vi "Get_Day_File_Data.vi"(4 "Use Full Res Files":bool, 5 "Averaging Time (min)":dbl=5.0, 6 "End time":timestamp, 7 "Start time":timestamp, 8 "Channel Names":string[](array[string])=["EnFlo Tun:Usonic Fixed:Velocity"], 9 "Data folder location":path) -> (0 "Files with wrong times":path[](array[path]), 1 "All Channel Names":string[](array[string]), 2 "Data":dbl[][](array[numeric]), 3 "Times":dbl[](array[numeric]))   [LabVIEW 2020]
uses:
  Anemometry/Anemometry Sub Vis/Globals/Constants_global.vi
  Anemometry/Anemometry Sub Vis/Globals/Preference_global.vi
panel:
  out "Currenly reading":path
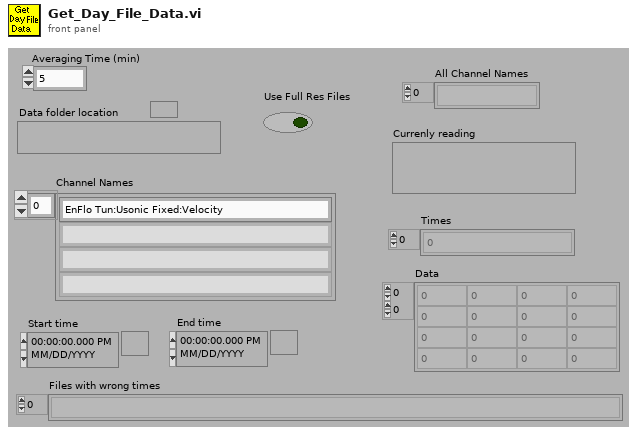
[diagram p1: front panel]
types:
  T1 = typedef "LVDateTimeRec.ctl" = cluster{"fractional second":dbl, "second":i32, "minute":i32, "hour":i32, "day of month":i32, "month":i32, "year":i32, "day of week":i32, "day of year":i32, "DST":i32}
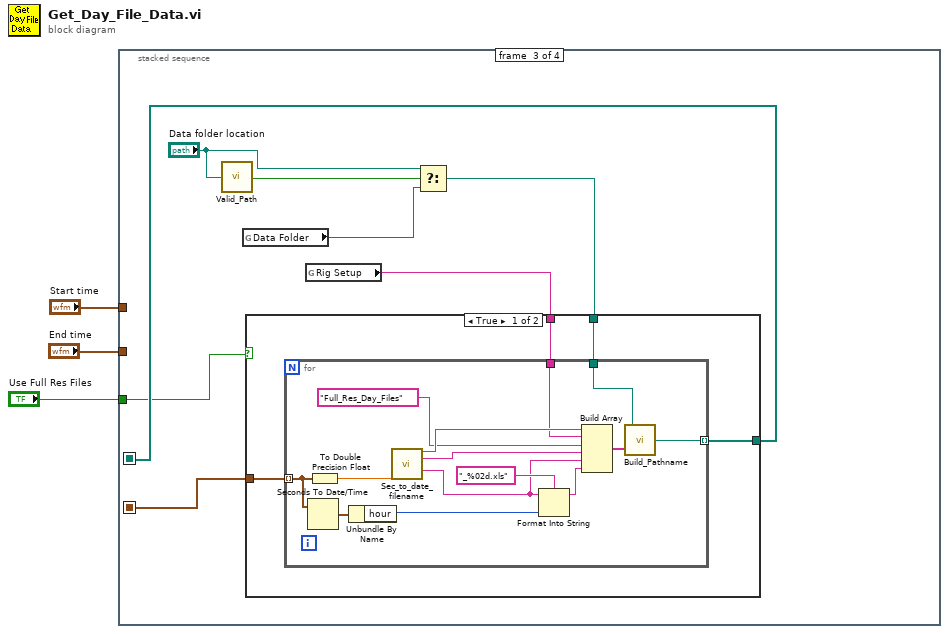
[diagram p0: block diagram]
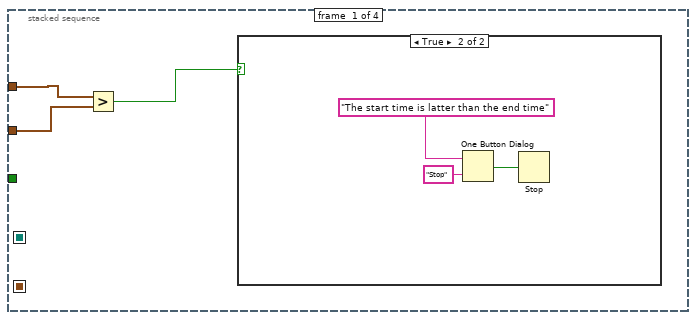
[diagram p2: hidden frame]
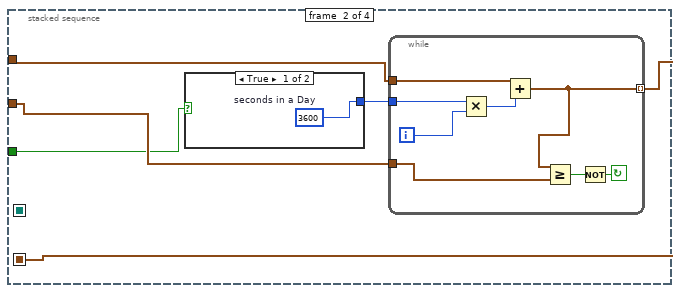
[diagram p4: hidden frame]
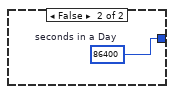
[diagram p5: hidden frame]
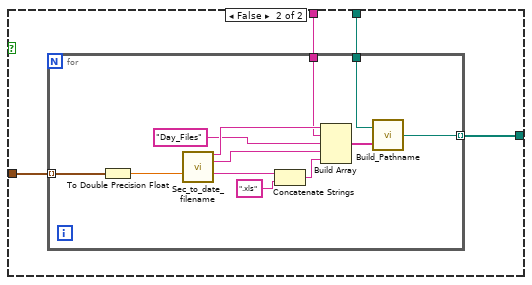
[diagram p6: hidden frame]
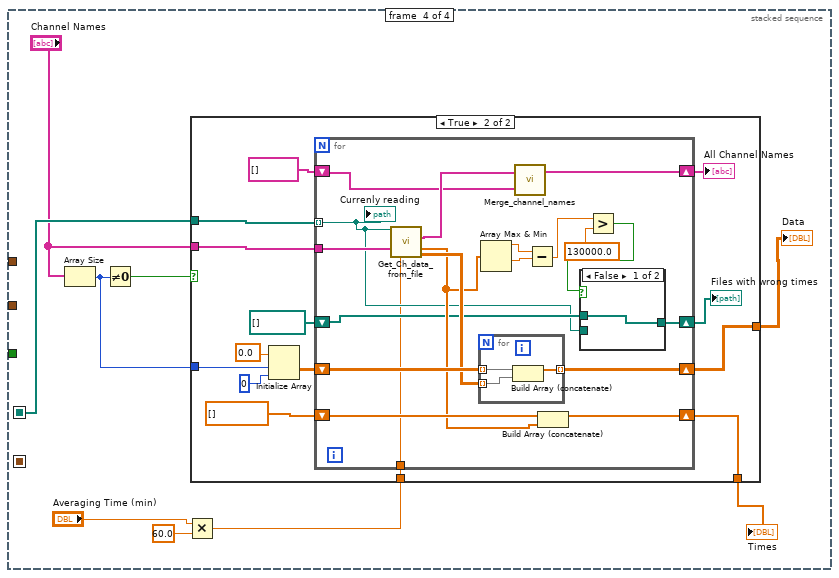
[diagram p7: hidden frame]
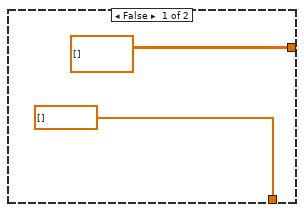
[diagram p8: hidden frame]
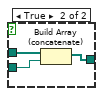
[diagram p9: hidden frame]
diagram:
  n1 = stacked-sequence {
    seq-local: [_ w14 _ _] -> [_ _ w32 _]
    seq-local: [_ _ w31 _] -> [_ _ _ w75]
    tunnel: "End time" -> [w5 w11 _ _]
    tunnel: "Start time" -> [w4 w12 _ _]
    tunnel: "Use Full Res Files" -> [_ w10 w25 _]
    frame #0 {
      n2 = Greater?(x=w4, y=w5) -> (0:w6:bool)
      n3 = case shown="True" w6 {
        frame False {
        }
        frame True {
          n4 = One Button Dialog(message="The start time is latter than the end time", button name ("OK")="Stop") -> (true=w8:bool)
          n5 = Stop(stop? (T)=w8) -> ()
        }
      }
    }
    frame #1 {
      n6 = case shown="True" w10 {
        tunnel: [w15 w16] -> w13
        frame True {
          w15 = u32 3600  # seconds in a Day
        }
        frame False {
          w16 = u32 86400  # seconds in a Day
        }
      }
      n7 = while {
        tunnel: [w17] -> w14 mode=indexing
        tunnel: w11 -> [w24]
        tunnel: w12 -> [w18]
        tunnel: w13 -> [w20]
        i -> [w21]
        stop <- w22 continue-if-true
        n8 = Multiply(x=w20, y=w21) -> (x*y=w19:u32)
        n9 = Add(x=w18, y=w19) -> (x+y=w17:timestamp)
        n10 = Greater Or Equal?(x=w17, y=w24) -> (x >= y?=w23:bool)
        n11 = Not(x=w23) -> (.not. x?=w22:bool)
      }
    }
    frame #2 {
      n12 = call "Valid_Path.vi"("Filename"="Data folder location") -> ("Valid Path?"=w30:bool)
      n13 = global read "Constants_global.vi" "Data Folder"() -> (w28:path)
      n14 = global read "Preference_global.vi" "Rig Setup"() -> (w26:string)
      n15 = Select(t="Data folder location", s=w30, f=w28) -> (s? t:f=w27:path)
      n16 = case shown="True" w25 {
        tunnel: w32 -> [w36 w54]
        tunnel: [w33 w53] -> w31
        tunnel: w27 -> [w35 w52]
        tunnel: w26 -> [w34 w51]
        frame True {
          n17 = for {
            tunnel: w36 -> [w44] mode=indexing
            tunnel: w35 -> [w46]
            tunnel: w34 -> [w47]
            tunnel: [w40] -> w33 mode=indexing
            n18 = Seconds To Date/Time(time stamp (now)=w44) -> (date time rec=w45:T1)  [unwired: 1 in]
            n19 = To Double Precision Float(number=w44) -> (double precision float=w48:dbl)
            n20 = Unbundle By Name(w45) -> ("hour"=w43:i32)
            n21 = call "Sec_to_date_filename.vi"("ss1904"=w48) -> ("YYYY"=w50:string, "mm-YYYY"=w37:string, "DD-mm-YYYY"=w38:string)  [unwired: 5 in, 7 out]
            n22 = Format Into String(format string="_%02d.xls", initial string=w38, w43) -> (resulting string=w39:string)  [unwired: 1 in, 1 out]
            n23 = Build Array(w50, w47, "Full_Res_Day_Files" ("Input Element"), w37, w38, w39) -> (w42:string[])
            n24 = call "Build_Pathname.vi"("PathElements"=w42, "PathnameIn"=w46) -> ("AppendedPath"=w40:path)
          }
        }
        frame False {
          n25 = for {
            tunnel: w54 -> [w66] mode=indexing
            tunnel: w52 -> [w60]
            tunnel: [w57] -> w53 mode=indexing
            tunnel: w51 -> [w56]
            n26 = To Double Precision Float(number=w66) -> (double precision float=w58:dbl)
            n27 = call "Sec_to_date_filename.vi"("ss1904"=w58) -> ("YYYY"=w62:string, "mm-YYYY"=w55:string, "DD-mm-YYYY"=w65:string)  [unwired: 5 in, 7 out]
            n28 = Concatenate Strings(w65, ".xls" ("string")) -> (w63:string)
            n29 = Build Array(w62, w56, "Day_Files" ("Input Element"), w55, w63) -> (w59:string[])
            n30 = call "Build_Pathname.vi"("PathElements"=w59, "PathnameIn"=w60) -> ("AppendedPath"=w57:path)
          }
        }
      }
    }
    frame #3 {
      n31 = Array Size(array="Channel Names") -> (size(s)=w73:i32)
      n32 = Not Equal To 0?(x=w73) -> (x != 0?=w74:bool)
      n33 = Multiply(x="Averaging Time (min)", y=60.0) -> (x*y=w67:dbl)
      n34 = case shown="True" w74 {
        tunnel: w75 -> [_ w91]
        tunnel: [dbl[] [] w89] -> w71
        tunnel: [dbl[][] [] w88] -> w70
        tunnel: "Channel Names" -> [_ w86]
        tunnel: w73 -> [_ w84]
        tunnel: w67 -> [_ w78]
        frame False {
        }
        frame True {
          n35 = Initialize Array(0.0, w84, 0 ("Dimension Size")) -> (w82:dbl[][])
          n36 = for {
            tunnel: w91 -> [w93] mode=indexing
            shift-right: [w109] -> w88
            shift-left: w82 -> [w110]
            shift-right: [w108] -> w89
            shift-left: dbl[] [] -> [w107]
            shift-right: [w103] -> w79
            shift-left: string[] [] ("Merged Channels") -> [w104]
            tunnel: w86 -> [w102]
            shift-right: [w94] -> w80
            shift-left: path[] [] -> [w95]
            tunnel: w78 -> [w92]
            n37 = call "Get_Ch_data_from_file.vi"("Filename"=w93, "Channel names"=w102, "Averaging Time(s)"=w92) -> ("File Channels"=w105:string[], "Times"=w101:dbl[], "Ch Data"=w106:dbl[][])  [unwired: 1 in, 9 out]
            n38 = for {
              tunnel: w110 -> [w117] mode=indexing
              tunnel: [w116] -> w109 mode=indexing
              tunnel: w106 -> [w115] mode=indexing
              n39 = Build Array (concatenate)(w117, w115) -> (w116:dbl[])
            }
            n40 = Array Max & Min(array=w101) -> (max value=w100:dbl, min value=w99:dbl)  [unwired: 2 out]
            n41 = call "Merge_channel_names.vi"("Preferred Channel array"=w105, "Channel array"=w104) -> ("Merged Channels"=w103:string[])  [unwired: 2 out]
            n42 = Subtract(x=w100, y=w99) -> (x-y=w98:dbl)
            n43 = Build Array (concatenate)(w107, w101) -> (w108:dbl[])
            n44 = Greater?(x=w98, y=130000.0) -> (0:w96:bool)
            n45 = case shown="False" w96 {
              tunnel: w95 -> [w111 w114]
              tunnel: [w111 w113] -> w94
              tunnel: w93 -> [_ w112]
              frame False {
              }
              frame True {
                n46 = Build Array (concatenate)(w114, w112) -> (w113:path[])
              }
            }
            "Currenly reading" <- w93
          }
          "Files with wrong times" <- w80
          "All Channel Names" <- w79
        }
      }
      "Times" <- w71
      "Data" <- w70
    }
  }
